vi "switch_get.vi"(7 "LabVIEW Web Service Request":refnum<class "Web Request.lvclass">) -> ()   [LabVIEW 2014]
uses:
  <vilib>/wsapi/Web Request.lvclass
  DataManager/StateStore/Controls/DataFunction.ctl
panel:
  out "error out 2":errorcluster
  out "timing":u32
  out "error out":errorcluster
  # "Use the Web Service Request input terminal to call the VIs on the Web Services palette. Do not remove it from the connector pane unless you don't need access to the palette."
  # "Each additional control wired to the connector pane will be available as an input in the URL. To include an indicator in terminal-mode output (the default setting), it must also be wired to the connector pane."
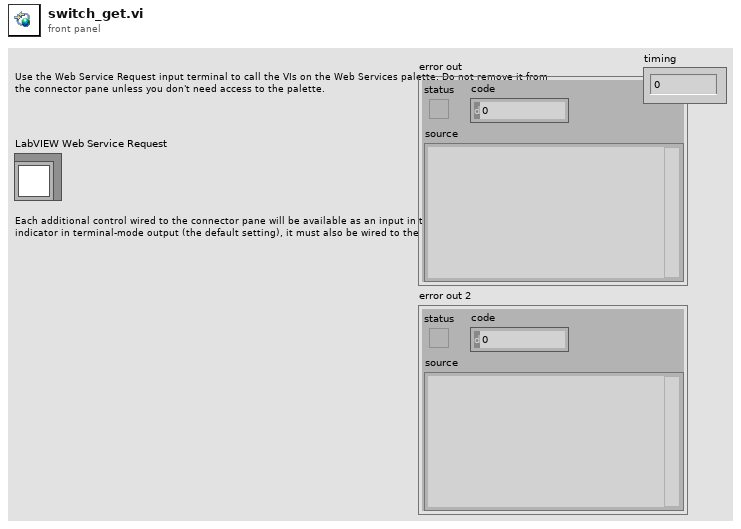
[diagram p1: front panel]
types:
  T1 = typedef "DataFunction.ctl" = enum16{"Initialise", "Release", "Get Data", "Set Data", "Preview Data"}
  T2 = typedef "CData Core Control.ctl" = cluster{"train_data_array":cluster{"uuid":string, "int":i32, "posit_array":cluster{"x":dbl, "y":dbl, "z":dbl}[]}[], "train_control_array":cluster{"uuid":string, "throttle":dbl, "brake":dbl, "horn":dbl, "wait":dbl, "name":string, "mode":string, "dest":string}[], "switch_data_array":cluster{"switch_posit":cluster{"x":dbl, "y":dbl, "z":dbl}, "manual":bool}[], "switch_control_array":cluster{"switch_posit":cluster{"x":dbl, "y":dbl, "z":dbl}, "switch":bool, "invert":bool, "wait":dbl}[]}
  T3 = cluster{"switch_posit":cluster{"x":dbl, "y":dbl, "z":dbl}, "switch":bool, "invert":bool, "wait":dbl}[]
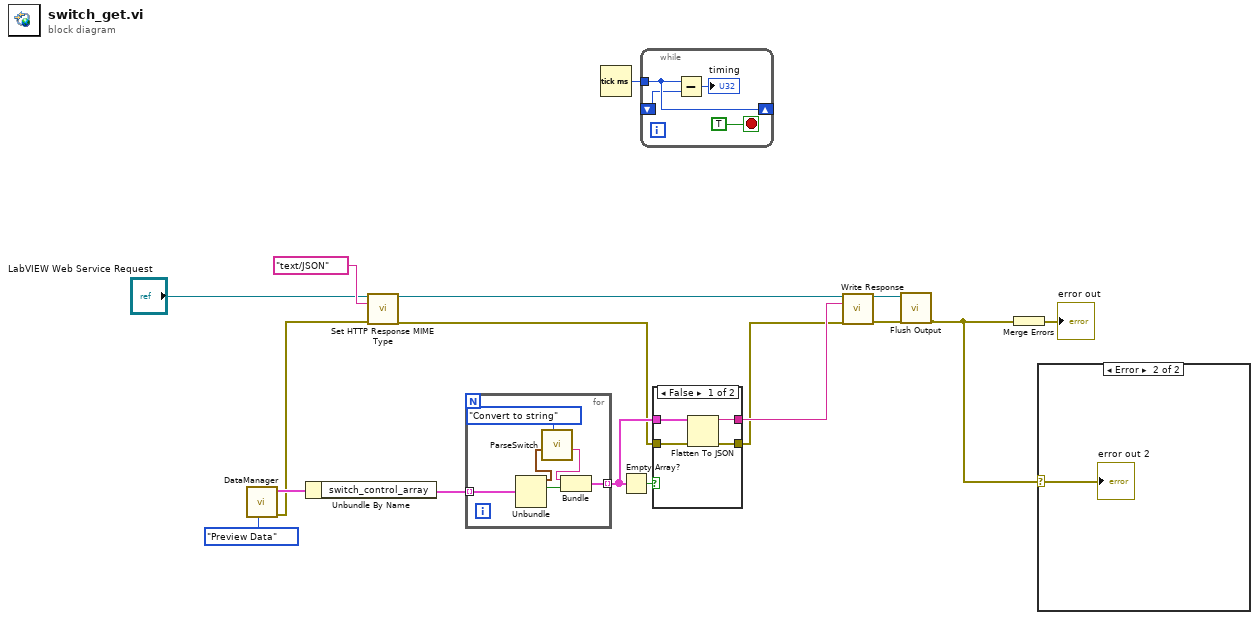
[diagram p0: block diagram]
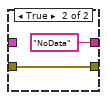
[diagram p2: hidden frame]
diagram:
  n1 = call "DataManager.vi"("DataFunction"=DataFunction."Preview Data") -> ("error out"=w11:errorcluster, "CData Out"=w12:T2)  [unwired: 9 in]
  n2 = Unbundle By Name(w12) -> ("switch_control_array"=w7:T3)
  n3 = call <vilib>:"Set HTTP Response MIME Type.vi"("LabVIEW Web Service Request"="LabVIEW Web Service Request", "MIME type (text/html)"="text/JSON", "error in (no error)"=w11) -> ("LabVIEW Web Service Request out"=w14:refnum<class "Web Request.lvclass">, "error out"=w5:errorcluster)  [unwired: 11 in]
  n4 = for {
    tunnel: w7 -> [w23] mode=indexing
    tunnel: [w21] -> w9 mode=indexing
    n5 = Unbundle(w23) -> ("switch_posit"=w19:cluster{"x":dbl, "y":dbl, "z":dbl}, "switch"=w22:bool)  [unwired: 2 out]
    n6 = call "ParseSwitch.vi"("Enum"=enum16{"Parse", "Convert to string"}."Convert to string", "cluster in"=w19) -> ("pos"=w18:string)  [unwired: 8 in, 1 out]
    n7 = Bundle("pos"=w18, "switch"=w22) -> (w21:cluster{"pos":string, "switch":bool})  [unwired: 1 in]
  }
  n8 = Tick Count (ms)() -> (millisecond timer value=w10:u32)
  n9 = Empty Array?(array=w9) -> (empty?=w8:bool)
  n10 = while {
    tunnel: w10 -> [w27]
    shift-right: [w27] -> _
    shift-left: _ -> [w26]
    stop <- TRUE stop-if-true
    n11 = Subtract(x=w27, y=w26) -> (x-y=→"timing":u32)
  }
  n12 = case shown="False" w8 {
    tunnel: [w28 "NoData" ("JSON string")] -> w6
    tunnel: w9 -> [w31 _]
    tunnel: w5 -> [w30 w33]
    tunnel: [w29 w33] -> w4
    frame False {
      n13 = Flatten To JSON(anything=w31, error in (no error)=w30) -> (JSON string=w28:string, 11:w29:errorcluster)  [unwired: 1 in]
    }
    frame True {
    }
  }
  n14 = call <vilib>:"Write Response.vi"("LabVIEW Web Service Request"=w14, "response string"=w6, "error in (no error)"=w4) -> ("LabVIEW Web Service Request out"=w3:refnum<class "Web Request.lvclass">, "error out"=w2:errorcluster)  [unwired: 11 in]
  n15 = call <vilib>:"Flush Output.vi"("LabVIEW Web Service Request"=w3, "error in (no error)"=w2) -> ("error out"=w1:errorcluster)  [unwired: 12 in, 1 out]
  n16 = Merge Errors(w1) -> (→"error out":errorcluster)
  n17 = case shown="Error" w1 {
    selector: w1 -> [_ w34]
    frame No Error {
    }
    frame Error {
      "error out 2" <- w34
    }
  }
